vi "Label_Prefix.vi"() -> (0 "Label Prefix String":string)   [LabVIEW 2016, in "CCD.lvlib" / "CCD Configuration.lvclass"]
uses:
  <userlib>/Common Components/Hardware/CCD/CCD Configuration.lvclass
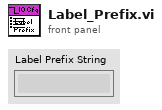
[diagram p1: front panel]
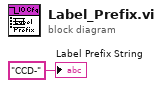
[diagram p0: block diagram]
diagram:
  "Label Prefix String" <- "CCD-" ("Label Prefix String")
